vi "Decompose LabVIEW Object - String - Private Data Cluster Value.vi"() -> ()   [LabVIEW 2017, in "Composition.Tests.lvlib"]
uses:
  Composition.Tests.lvlib
  Classes/String/String.lvclass
  Composition/Composition.lvlib
  <vilib>/addons/_JKI Toolkits/Caraya/classes/Test/Test.lvclass
  <vilib>/addons/_JKI Toolkits/Caraya/classes/Assert/Assert.lvclass
panel:
  out "error out":errorcluster
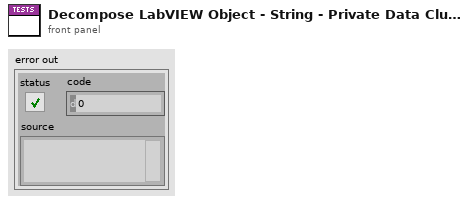
[diagram p1: front panel]
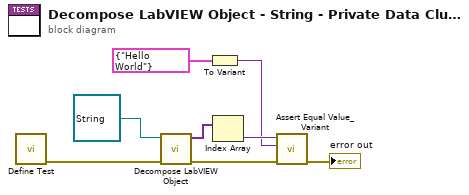
[diagram p0: block diagram]
diagram:
  n1 = call <vilib>:"Define Test.vi"() -> ("error out"=w3:errorcluster)  [unwired: 11 in]
  n2 = call "Decompose LabVIEW Object.vi"("error in (no error)"=w3, "LabVIEW Object"=refnum<class "String.lvclass"> refnum ("Reflection.Tests.lvlib:String.lvclass")) -> ("error out"=w7:errorcluster, "Private Data Clusters"=w5:variant[])  [unwired: 6 in, 2 out]
  n3 = To Variant(anything=cluster{string} {"Hello World"}) -> (Variant=w1:variant)
  n4 = Index Array(array=w5) -> (element=w2:variant)  [unwired: 1 in]
  n5 = call <vilib>:"Assert Equal Value_Variant.vi"("error in (no error)"=w7, "Y"=w1, "X"=w2) -> ("error out"=→"error out":errorcluster)  [unwired: 8 in]
